vi "ALTS-2015 Write Robot on OPC v0.1.vi"(7 "Option":T1=enum."Write Invalid Serial Task", 8 "error in (no error)":errorcluster, 10 "Station # Load":T2, 11 "Serial Details in":T3) -> (0 "error out":errorcluster)   [LabVIEW 2013]
uses:
  OPC Engine/Controls/ALTS-2015 OPC Write Global Options.ctl
  OPC Engine/Controls/ALTS-2015 OPC Write Registers.ctl
  Controls/ALTS-2015 Task at Station Options.ctl
  Controls/ALTS-2015 Station Cluster.ctl
  Controls/ALTS-2015 Serial Details.ctl
  Controls/ALTS-2015 Write Robot Task OPC Options.ctl
  Controls/ALTS-2015 Serial DB Details.ctl
  Controls/ALTS-2015 Robot Tasks.ctl
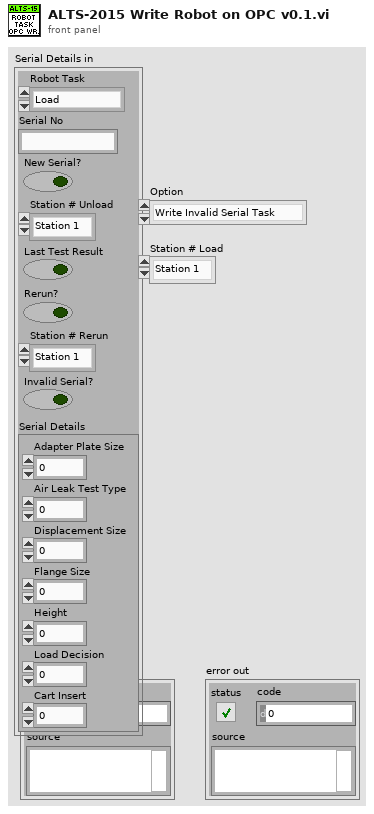
[diagram p1: front panel]
types:
  T1 = typedef "ALTS-2015 Write Robot Task OPC Options.ctl" = enum16{"Write New Serial Task", "Write Rerun Task", "Write Unload Task", "Write Invalid Serial Task"}
  T2 = typedef "ALTS-2015 Station Cluster.ctl" = enum16{"Station 1", "Station 2", "Station 3", "Station 4"}
  T3 = typedef "ALTS-2015 Serial Details.ctl" = cluster{"Robot Task":T4, "Serial No":string, "New Serial?":bool, "Station # Unload":T2, "Last Test Result":bool, "Rerun?":bool, "Station # Rerun":T2, "Invalid Serial?":bool, "Serial Details":T5}
  T4 = typedef "ALTS-2015 Robot Tasks.ctl" = enum16{"Load", "Unload", "Rerun", "Invalid Serial"}
  T5 = typedef "ALTS-2015 Serial DB Details.ctl" = cluster{"Adapter Plate Size":i32, "Air Leak Test Type ":i32, "Displacement Size":i32, "Flange Size":i32, "Height":i32, "Load Decision":i32, "Cart Insert":i32}
  T6 = typedef "ALTS-2015 Task at Station Options.ctl" = enum16{"Init", "Write", "Read All", "Read"}
  T7 = typedef "ALTS-2015 OPC Write Global Options.ctl" = enum16{"Init", "Write Value", "Write Array", "Read Value", "Read Array", "Read All"}
  T8 = typedef "ALTS-2015 OPC Write Registers.ctl" = enum16{"Task_Available_for_Robot", "New_Serial", "Serial_Adapter_Size", "Serial_Displacement_Size", "Serial_Flange_Size", "Serial_Height", "Serial_LoadDecision", "Serial_CartInsert", "Test_Result", "Station_Number", "Rerun", "Invalid_SNo", "PC_ACK_Read_Tags", "No_Test"}
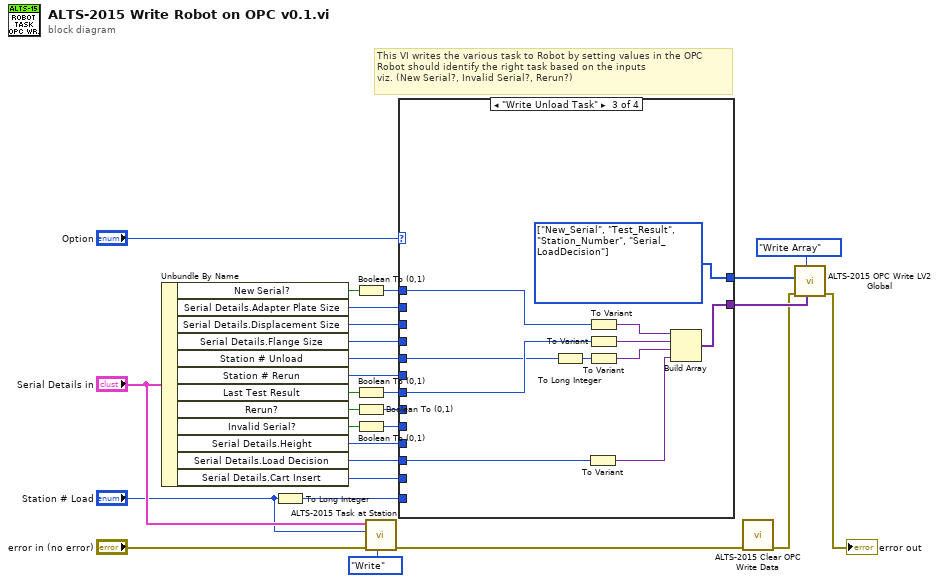
[diagram p0: block diagram]
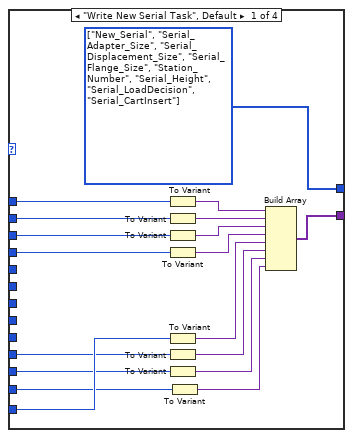
[diagram p2: hidden frame]
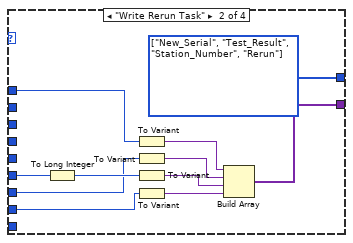
[diagram p3: hidden frame]
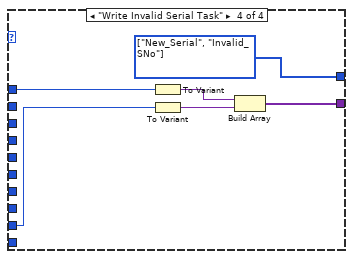
[diagram p4: hidden frame]
diagram:
  # "This VI writes the various task to Robot by setting values in the OPC\nRobot should identify the right task based on the inputs \nviz. (New Serial?, Invalid Serial?, Rerun?)"
  n1 = Unbundle By Name("Serial Details in") -> ("New Serial?"=w23:bool, "Serial Details.Adapter Plate Size"=w24:i32, "Serial Details.Displacement Size"=w25:i32, "Serial Details.Flange Size"=w27:i32, "Station # Unload"=w16:T2, "Station # Rerun"=w17:T2, "Last Test Result"=w18:bool, "Rerun?"=w15:bool, "Invalid Serial?"=w19:bool, "Serial Details.Height"=w8:i32, "Serial Details.Load Decision"=w7:i32, "Serial Details.Cart Insert"=w6:i32)
  n2 = To Long Integer(number="Station # Load") -> (32bit integer=w3:i32)
  n3 = Boolean To (0,1)(Boolean=w23) -> (0, 1=w12:i16)
  n4 = Boolean To (0,1)(Boolean=w18) -> (0, 1=w13:i16)
  n5 = Boolean To (0,1)(Boolean=w15) -> (0, 1=w11:i16)
  n6 = Boolean To (0,1)(Boolean=w19) -> (0, 1=w10:i16)
  n7 = call "ALTS-2015 Task at Station.vi"("Options"=ALTS-2015_Task_at_Station_Options."Write", "error in (no error)"="error in (no error)", "Station # Load"="Station # Load", "Serial Details in"="Serial Details in") -> ("error out"=w4:errorcluster)  [unwired: 5 in, 2 out]
  n8 = case shown="\"Write Unload Task\"" "Option" {
    tunnel: [w46 w51 w64 w71] -> w14
    tunnel: w27 -> [w45 _ _ _]
    tunnel: [w44 w52 w63 w72] -> w26
    tunnel: w25 -> [w43 _ _ _]
    tunnel: w24 -> [w42 _ _ _]
    tunnel: w12 -> [w41 w50 w62 w69]
    tunnel: w10 -> [_ _ _ w70]
    tunnel: w13 -> [_ w49 w61 _]
    tunnel: w17 -> [_ w48 _ _]
    tunnel: w16 -> [_ _ w59 _]
    tunnel: w11 -> [_ w47 _ _]
    tunnel: w3 -> [w35 _ _ _]
    tunnel: w8 -> [w33 _ _ _]
    tunnel: w7 -> [w31 _ w58 _]
    tunnel: w6 -> [w30 _ _ _]
    frame "Write New Serial Task", Default {
      w44 = T8[] [enum."New_Serial", enum."Serial_Adapter_Size", enum."Serial_Displacement_Size", enum."Serial_Flange_Size", enum."Station_Number", enum."Serial_Height", enum."Serial_LoadDecision", enum."Serial_CartInsert"] items=["Task_Available_for_Robot", "New_Serial", "Serial_Adapter_Size", "Serial_Displacement_Size", "Serial_Flange_Size", "Serial_Height", "Serial_LoadDecision", "Serial_CartInsert", "Test_Result", "Station_Number", "Rerun", "Invalid_SNo", "PC_ACK_Read_Tags", "No_Test"] ("OPC Write Register Array")
      n9 = To Variant(anything=w41) -> (Variant=w40:variant)
      n10 = To Variant(anything=w42) -> (Variant=w39:variant)
      n11 = To Variant(anything=w43) -> (Variant=w38:variant)
      n12 = To Variant(anything=w45) -> (Variant=w37:variant)
      n13 = To Variant(anything=w35) -> (Variant=w36:variant)
      n14 = To Variant(anything=w33) -> (Variant=w34:variant)
      n15 = To Variant(anything=w31) -> (Variant=w32:variant)
      n16 = To Variant(anything=w30) -> (Variant=w29:variant)
      n17 = Build Array(w40, w39, w38, w37, w36, w34, w32, w29) -> (w46:variant[])
    }
    frame "Write Rerun Task" {
      w52 = T8[] [enum."New_Serial", enum."Test_Result", enum."Station_Number", enum."Rerun"] items=["Task_Available_for_Robot", "New_Serial", "Serial_Adapter_Size", "Serial_Displacement_Size", "Serial_Flange_Size", "Serial_Height", "Serial_LoadDecision", "Serial_CartInsert", "Test_Result", "Station_Number", "Rerun", "Invalid_SNo", "PC_ACK_Read_Tags", "No_Test"] ("OPC Write Register Array")
      n18 = To Long Integer(number=w48) -> (32bit integer=w53:i32)
      n19 = To Variant(anything=w50) -> (Variant=w57:variant)
      n20 = To Variant(anything=w49) -> (Variant=w56:variant)
      n21 = To Variant(anything=w53) -> (Variant=w55:variant)
      n22 = To Variant(anything=w47) -> (Variant=w54:variant)
      n23 = Build Array(w57, w56, w55, w54) -> (w51:variant[])
    }
    frame "Write Unload Task" {
      w63 = T8[] [enum."New_Serial", enum."Test_Result", enum."Station_Number", enum."Serial_LoadDecision"] items=["Task_Available_for_Robot", "New_Serial", "Serial_Adapter_Size", "Serial_Displacement_Size", "Serial_Flange_Size", "Serial_Height", "Serial_LoadDecision", "Serial_CartInsert", "Test_Result", "Station_Number", "Rerun", "Invalid_SNo", "PC_ACK_Read_Tags", "No_Test"] ("OPC Write Register Array")
      n24 = To Long Integer(number=w59) -> (32bit integer=w65:i32)
      n25 = To Variant(anything=w58) -> (Variant=w60:variant)
      n26 = To Variant(anything=w62) -> (Variant=w68:variant)
      n27 = To Variant(anything=w61) -> (Variant=w67:variant)
      n28 = To Variant(anything=w65) -> (Variant=w66:variant)
      n29 = Build Array(w68, w67, w66, w60) -> (w64:variant[])
    }
    frame "Write Invalid Serial Task" {
      w72 = T8[] [enum."New_Serial", enum."Invalid_SNo"] items=["Task_Available_for_Robot", "New_Serial", "Serial_Adapter_Size", "Serial_Displacement_Size", "Serial_Flange_Size", "Serial_Height", "Serial_LoadDecision", "Serial_CartInsert", "Test_Result", "Station_Number", "Rerun", "Invalid_SNo", "PC_ACK_Read_Tags", "No_Test"] ("OPC Write Register Array")
      n30 = To Variant(anything=w69) -> (Variant=w74:variant)
      n31 = To Variant(anything=w70) -> (Variant=w73:variant)
      n32 = Build Array(w74, w73) -> (w71:variant[])
    }
  }
  n33 = call "ALTS-2015 Clear OPC Write Data.vi"("error in (no error)"=w4) -> ("error out"=w9:errorcluster)  [unwired: 10 in]
  n34 = call "ALTS-2015 OPC Write LV2 Global.vi"("OPC value Array"=w14, "Options"=ALTS-2015_OPC_Write_Global_Options."Write Array", "error in (no error)"=w9, "OPC Write Register Array"=w26) -> ("error out"=→"error out":errorcluster)  [unwired: 5 in, 2 out]
